vi "Compare Folder Shots.vi"(8 "error in (no error)":errorcluster, 10 "Folder Shot 2":T1[](array[typedef]), 11 "Folder Shot 1":T1[](array[typedef])) -> (0 "error out":errorcluster, 1 "Files Deleted":path[](array[path]), 2 "Files Added":path[](array[path]), 3 "Files Modified":path[](array[path]))   [LabVIEW 2014, in "SLL File IO.lvlib"]
doc: "Compare two FolderShot Clusters."
uses:
  SLL File IO.lvlib
  _Typedefs/Folder Shot Element.ctl
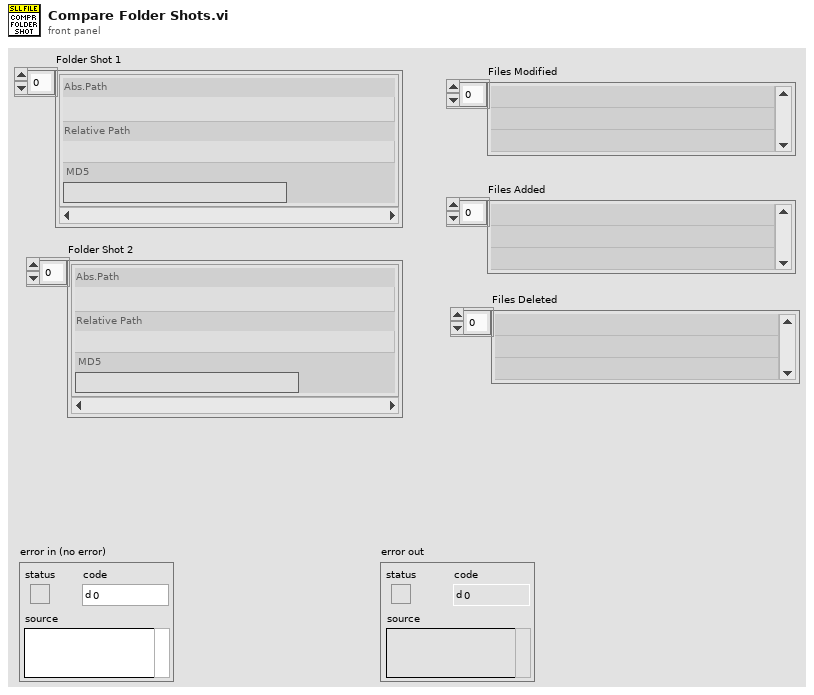
[diagram p1: front panel]
types:
  T1 = typedef "SLL File IO.lvlib/Folder Shot Element.ctl" = cluster{"Abs.Path":path, "Relative Path":path, "MD5":string}
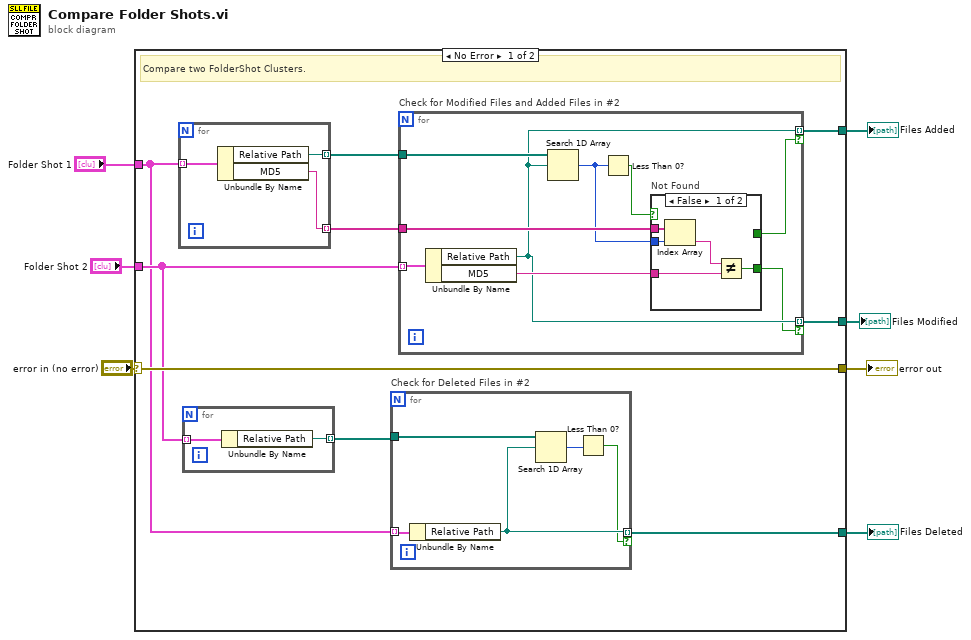
[diagram p0: block diagram]
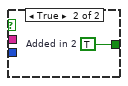
[diagram p2: hidden frame]
diagram:
  n1 = case shown="No Error" "error in (no error)" {
    selector: "error in (no error)" -> [w16 w42]
    tunnel: [w16 w42] -> w6
    tunnel: "Folder Shot 1" -> [w10 _]
    tunnel: "Folder Shot 2" -> [w11 _]
    tunnel: [w13 _] -> w3
    tunnel: [w12 _] -> w2
    tunnel: [w8 _] -> w1
    frame No Error {
      # "Compare two FolderShot Clusters."
      n2 = for {
        tunnel: w10 -> [w41] mode=indexing
        tunnel: [w40] -> w15 mode=indexing
        tunnel: [w39] -> w14 mode=indexing
        n3 = Unbundle By Name(w41) -> ("Relative Path"=w40:path, "MD5"=w39:string)
      }
      n4 = for {
        tunnel: w11 -> [w23] mode=indexing
        tunnel: [w22] -> w9 mode=indexing
        n5 = Unbundle By Name(w23) -> ("Relative Path"=w22:path)
      }
      n6 = for "Check for Deleted Files in #2" {
        tunnel: w10 -> [w20] mode=indexing
        tunnel: w9 -> [w21]
        tunnel: [w18] -> w8 mode=indexing if=w17
        n7 = Unbundle By Name(w20) -> ("Relative Path"=w18:path)
        n8 = Search 1D Array(1D array=w21, element=w18) -> (index of element=w19:i32)  [unwired: 1 in]
        n9 = Less Than 0?(x=w19) -> (x < 0?=w17:bool)
      }
      n10 = for "Check for Modified Files and Added Files in #2" {
        tunnel: w11 -> [w32] mode=indexing
        tunnel: w15 -> [w31]
        tunnel: w14 -> [w30]
        tunnel: [w26] -> w12 mode=indexing if=w24
        tunnel: [w26] -> w13 mode=indexing if=w25
        n11 = Unbundle By Name(w32) -> ("Relative Path"=w26:path, "MD5"=w29:string)
        n12 = Search 1D Array(1D array=w31, element=w26) -> (index of element=w28:i32)  [unwired: 1 in]
        n13 = Less Than 0?(x=w28) -> (x < 0?=w27:bool)
        n14 = case "Not Found" shown="False" w27 {
          tunnel: w30 -> [w37 _]
          tunnel: w29 -> [w35 _]
          tunnel: w28 -> [w34 _]
          tunnel: [w33 _] -> w25
          tunnel: [_ w38] -> w24
          frame False {
            n15 = Index Array(array=w37, index=w34) -> (element=w36:string)
            n16 = Not Equal?(x=w36, y=w35) -> (x != y?=w33:bool)
          }
          frame True {
            w38 = TRUE  # Added in 2
          }
        }
      }
    }
    frame Error {
    }
  }
  "error out" <- w6
  "Files Modified" <- w3
  "Files Added" <- w2
  "Files Deleted" <- w1
